vi "Query File List.vi"(8 "error in (no error)":errorcluster, 11 "VISA resource name":refnum<visa-resource-name>) -> (0 "error out":errorcluster, 1 "Memory Free":i32, 2 "Memory Used":i32, 3 "VISA resource name out":refnum<visa-resource-name>, 4 "File List":T1(array[cluster]))   [LabVIEW 2013, in "Agilent 3446X Series.lvlib"]
doc: "Returns a list of files in the specified folder."
uses:
  Agilent 3446X Series.lvlib
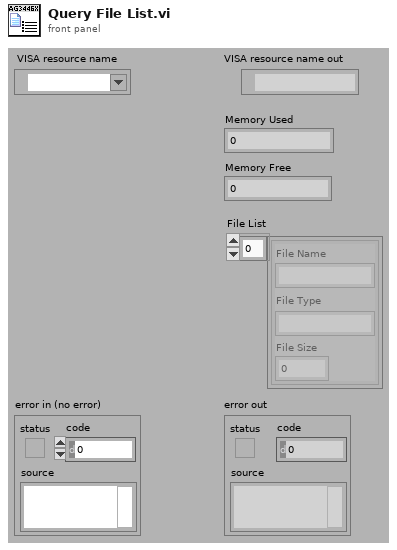
[diagram p1: front panel]
types:
  T1 = cluster{"File Name":string, "File Type":string, "File Size":i32}[]
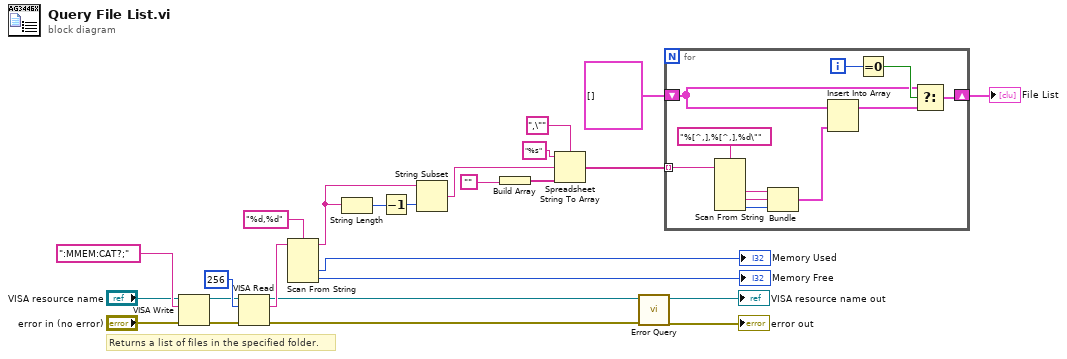
[diagram p0: block diagram]
diagram:
  # "Returns a list of files in the specified folder."
  n1 = VISA Write(VISA resource name="VISA resource name", write buffer=":MMEM:CAT?;", error in (no error)="error in (no error)") -> (VISA resource name out=w19:refnum<visa-resource-name>, error out=w18:errorcluster)  [unwired: 1 out]
  n2 = VISA Read(VISA resource name=w19, byte count=u32 256, error in (no error)=w18) -> (VISA resource name out=w13:refnum<visa-resource-name>, read buffer=w17:string, error out=w12:errorcluster)  [unwired: 1 out]
  n3 = Scan From String(format string="%d,%d", input string=w17) -> (remaining string=w11:string, output 1=→"Memory Used":i32, output 2=→"Memory Free":i32)  [unwired: 2 in, 4 out]
  n4 = String Length(string=w11) -> (length=w10:i32)
  n5 = Decrement(x=w10) -> (x-1=w9:i32)
  n6 = String Subset(string=w11, length (rest)=w9) -> (substring=w8:string)  [unwired: 1 out]
  n7 = Build Array("") -> (w6:string[])
  n8 = Spreadsheet String To Array(delimiter (Tab)=",\"", format string="%s", spreadsheet string=w8, array type (2D Dbl)=w6) -> (array=w2:string[])
  n9 = call "Error Query.vi"("error in (no error)"=w12, "VISA resource name"=w13) -> ("error out"=→"error out":errorcluster, "VISA resource name out"=→"VISA resource name out":refnum<visa-resource-name>)  [unwired: 8 out]
  n10 = for {
    tunnel: w2 -> [w26] mode=indexing
    shift-right: [w27] -> w1
    shift-left: T1 [] ("File List") -> [w29]
    i -> [w31]
    n11 = Scan From String(format string="%[^,],%[^,],%d\"", input string=w26) -> (output 1=w35:string, output 2=w34:string, output 3=w33:i32)  [unwired: 2 in, 6 out]
    n12 = Bundle(w35, w34, w33) -> (w32:cluster{string, string, i32})  [unwired: 1 out]
    n13 = Insert Into Array(array=w29, new element=w32) -> (w28:T1)  [unwired: 1 in]
    n14 = Equal To 0?(x=w31) -> (x = 0?=w30:bool)
    n15 = Select(t=w29, s=w30, f=w28) -> (s? t:f=w27:T1)
  }
  "File List" <- w1
